vi "MouseDown Response.vi"(4 "PlatMods":T1, 6 "Mods":cluster{"Double Click":bool, "Menu Key":bool}, 8 "error in (no error)":errorcluster, 9 "Button":u16, 10 "Coords":T2, 11 "Editor Handler in":refnum<class "3DButton Handler.lvclass">) -> (0 "error out":errorcluster, 3 "Editor Handler out":refnum<class "3DButton Handler.lvclass">)   [LabVIEW 2016, in "3DButton Handler.lvclass"]
uses:
  3DButton Handler.lvclass
  C:/Program Files (x86)/National Instruments/LabVIEW 2016/vi.lib/LIEF/Image Editor Handler/Image Editor Handler.lvclass
  <vilib>/Utility/miscctls.llb/LVPoint32TypeDef.ctl
  <vilib>/LIEF/Image Editor Handler/Image Editor Handler.lvclass/Image Editor Handler.ctl
  Rectangle3D/Rectangle3D.lvclass
  C:/Program Files (x86)/National Instruments/LabVIEW 2016/vi.lib/LIEF/Forms/Shape/Shape.lvclass
  <vilib>/LIEF/Forms/Selection/Selection.lvclass
  <vilib>/LIEF/Forms/Selection/Selection.lvclass/Selection.ctl
  Rectangle3D/Rectangle3D.lvclass/Rectangle3D.ctl
  Rectangle3D/Write Clicked.vi
  <vilib>/LIEF/Forms/Selection/Read Selected Shape.vi
  <vilib>/LIEF/Image Editor Handler/Write Shapes.vi
  <vilib>/LIEF/Image Editor Handler/Read PictureRef.vi
  <vilib>/LIEF/Image Editor Handler/Read Shapes.vi
  <vilib>/LIEF/Forms/Shape/Shape.lvclass
  <vilib>/LIEF/Image Editor Handler/Image Editor Handler.lvclass
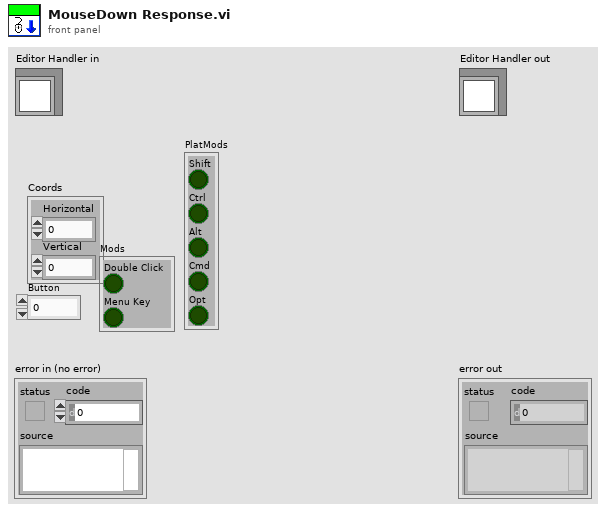
[diagram p1: front panel]
types:
  T1 = cluster{"Shift":bool, "Ctrl":bool, "Alt":bool, "Cmd":bool, "Opt":bool}
  T2 = typedef "LVPoint32TypeDef.ctl" = cluster{"Horizontal":i32, "Vertical":i32}
  T3 = typedef "LVPositionTypeDef.ctl" = cluster{"Left":i32, "Top":i32}
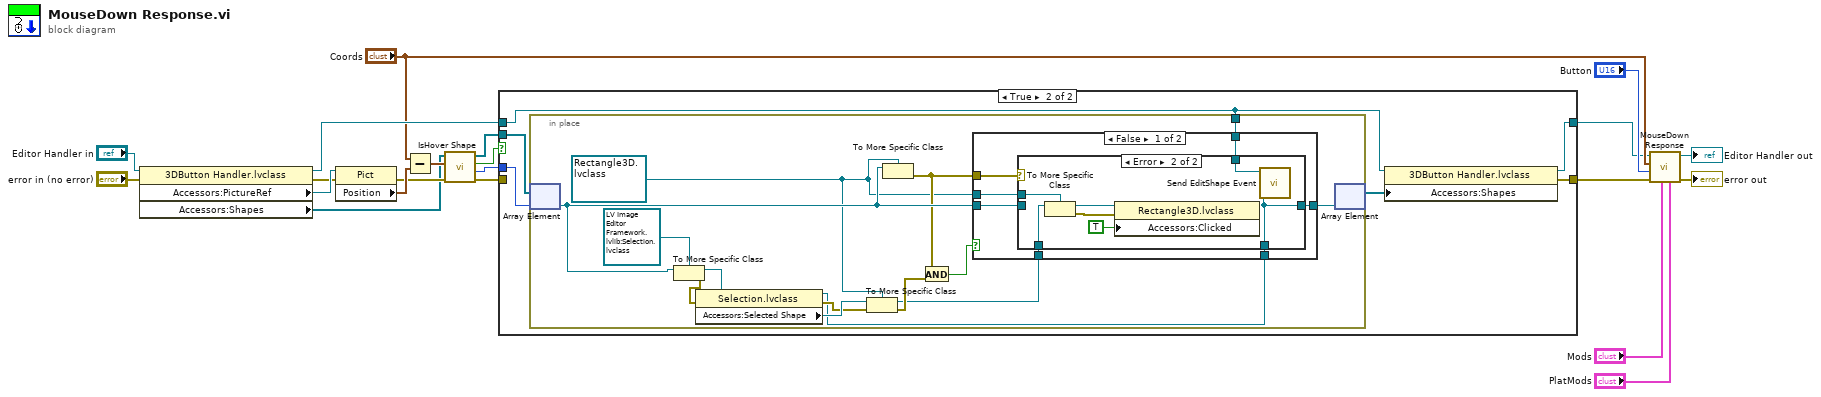
[diagram p0: block diagram]
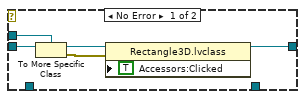
[diagram p3: hidden frame]
diagram:
  n1 = property class="3DButton Handler.lvclass"(reference="Editor Handler in", error in="error in (no error)") -> (reference out=w13:refnum<class "3DButton Handler.lvclass">, error out=w8:errorcluster, "Accessors:PictureRef"=w15:refnum<vi>, "Accessors:Shapes"=w14:refnum<data-value>[])
  n2 = property class="Pict"(reference=w15, error in=w8) -> (error out=w16:errorcluster, "Position"=w18:T3)  [unwired: 1 out]
  n3 = Subtract(x="Coords", y=w18) -> (x-y=w17:T2)
  n4 = call <vilib>:"IsHover Shape.vi"("error in (no error)"=w16, "Coords"=w17, "Shape in"=w14) -> ("error out"=w9:errorcluster, "Node ID"=w11:i32, "Found?"=w10:bool, "Shape out"=w12:refnum<data-value>[])  [unwired: 3 in, 2 out]
  n5 = case shown="True" w10 {
    tunnel: w13 -> [w23 w24]
    tunnel: w12 -> [_ w29]
    tunnel: w11 -> [_ w28]
    tunnel: [w23 w26] -> w5
    tunnel: [w22 w25] -> w3
    tunnel: w9 -> [w22 _]
    frame False {
    }
    frame True {
      n6 = in-place {
        in-place-border: w24 -> [w30]
        w35 = refnum<data-value> refnum ("target class")
        n7 = in-place-array #1(w29, w28) -> (w41:refnum<data-value>)
        n8 = To More Specific Class(target class=refnum<data-value> refnum, reference=w41) -> (specific class reference=w38:refnum<data-value>, error out=w34:errorcluster)  [unwired: 1 in]
        n9 = property class="Selection.lvclass"(reference=w38, error in=w34) -> (reference out=w31:refnum<data-value>, error out=w36:errorcluster, "Accessors:Selected Shape"=w37:refnum<data-value>)
        n10 = To More Specific Class(target class=w35, reference=w37, error in=w36) -> (specific class reference=w32:refnum<data-value>, error out=w33:errorcluster)
        n11 = To More Specific Class(target class=w35, reference=w41) -> (error out=w39:errorcluster)  [unwired: 1 in, 1 out]
        n12 = And(x=w39, y=w33) -> (x .and. y?=w40:bool)
        n13 = case shown="False" w40 {
          tunnel: [w50 w64] -> w43
          tunnel: w41 -> [w49 w64]
          tunnel: w35 -> [w48 _]
          tunnel: w39 -> [w47 _]
          tunnel: w32 -> [w46 _]
          tunnel: w31 -> [w45 _]
          tunnel: w30 -> [w44 _]
          frame False {
            n14 = case shown="Error" w47 {
              tunnel: [w56 w57] -> w50
              tunnel: w49 -> [w54 _]
              tunnel: w48 -> [w53 w62]
              tunnel: w46 -> [_ w59]
              tunnel: w45 -> [_ w57]
              tunnel: w44 -> [_ w58]
              frame No Error {
                n15 = To More Specific Class(target class=w53, reference=w54) -> (specific class reference=w52:refnum<data-value>, error out=w55:errorcluster)  [unwired: 1 in]
                n16 = property class="Rectangle3D.lvclass"(reference=w52, error in=w55, "Accessors:Clicked"=TRUE ("Clicked")) -> (reference out=w56:refnum<data-value>)  [unwired: 1 out]
              }
              frame Error {
                n17 = To More Specific Class(target class=w62, reference=w59) -> (specific class reference=w61:refnum<data-value>, error out=w63:errorcluster)  [unwired: 1 in]
                n18 = property class="Rectangle3D.lvclass"(reference=w61, error in=w63, "Accessors:Clicked"=TRUE ("Clicked")) -> ()  [unwired: 2 out]
                n19 = call <vilib>:"Send EditShape Event.vi"("Shape"=w57, "Editor Handler in"=w58) -> ()  [unwired: 8 in, 2 out]
              }
            }
          }
          frame True {
          }
        }
        n20 = in-place-array #1(w43) -> (w27:refnum<data-value>[])  [unwired: 1 out]
      }
      n21 = property class="3DButton Handler.lvclass"(reference=w24, "Accessors:Shapes"=w27) -> (reference out=w26:refnum<class "3DButton Handler.lvclass">, error out=w25:errorcluster)  [unwired: 1 in]
    }
  }
  n22 = call-parent "MouseDown Response.vi"("PlatMods"="PlatMods", "Mods"="Mods", "error in (no error)"=w3, "Button"="Button", "Coords"="Coords", "Editor Handler in"=w5) -> ("error out"=→"error out":errorcluster, "Editor Handler out"=→"Editor Handler out":refnum<class "3DButton Handler.lvclass">)  [unwired: 4 in]
